vi "Add Overall Status.vi"(8 "error in (no error)":errorcluster, 9 "Overall Status":string, 11 "Serial Number":string) -> (0 "error out":errorcluster)   [LabVIEW 2023, in "CSV Report.lvlib"]
uses:
  <vilib>/Utility/file.llb/Read Delimited Spreadsheet (string).vi
  <vilib>/Utility/file.llb/Write Delimited Spreadsheet (string).vi
  CSV Report.lvlib
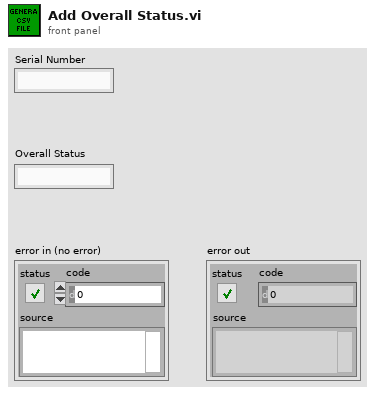
[diagram p1: front panel]
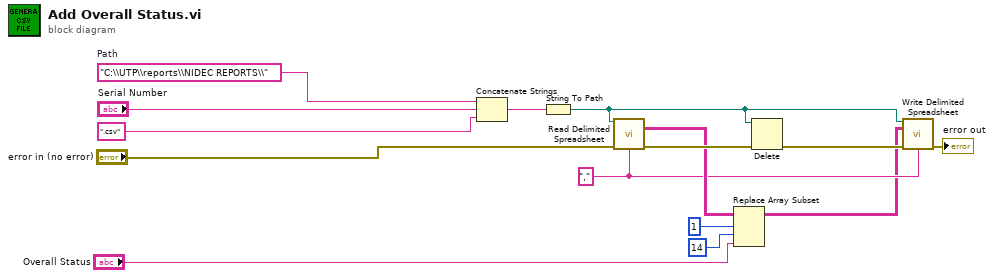
[diagram p0: block diagram]
diagram:
  w12 = "C:\\UTP\\reports\\NIDEC REPORTS\\"  # Path
  w5 = "," ("delimiter (\\t)")
  n1 = Concatenate Strings(w12, "Serial Number", ".csv" ("string")) -> (w11:string)
  n2 = String To Path(string=w11) -> (path=w4:path)
  n3 = call-poly <vilib>:"Read Delimited Spreadsheet.vi"("file path (dialog if empty)"=w4, "error in (no error)"="error in (no error)", "delimiter (\\t)"=w5) -> ("all rows"=w7:string[][], "error out"=w8:errorcluster)  [unwired: 7 in, 4 out]
  n4 = Replace Array Subset(array=w7, new element="Overall Status", index (row)=1, index (col)=14 ("disabled index (col)")) -> (w3:string[][])
  n5 = Delete(path (use dialog)=w4, error in=w8) -> (error out=w6:errorcluster)  [unwired: 3 in, 2 out]
  n6 = call-poly <vilib>:"Write Delimited Spreadsheet.vi"("file path (dialog if empty)"=w4, "2D data"=w3, "error in (no error)"=w6, "delimiter (\\t)"=w5) -> ("error out"=→"error out":errorcluster)  [unwired: 10 in, 1 out]
